vi "String to array.vi"(11 "String":string) -> (2 "Array":dbl[][](array[numeric]))   [LabVIEW 2016]
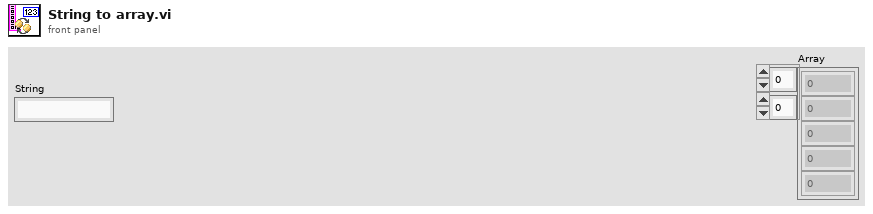
[diagram p1: front panel]
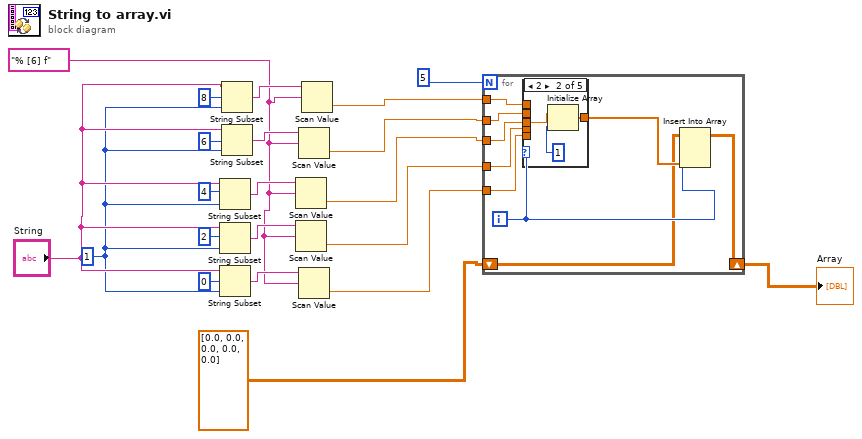
[diagram p0: block diagram]
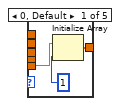
[diagram p2: hidden frame]
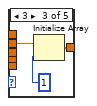
[diagram p3: hidden frame]
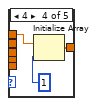
[diagram p4: hidden frame]
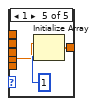
[diagram p5: hidden frame]
diagram:
  w1 = "% [6] f"
  w20 = 1
  n1 = String Subset(string="String", offset (0)=4, length (rest)=w20) -> (substring=w11:string)
  n2 = String Subset(string="String", offset (0)=2, length (rest)=w20) -> (substring=w10:string)
  n3 = String Subset(string="String", offset (0)=0, length (rest)=w20) -> (substring=w8:string)
  n4 = String Subset(string="String", offset (0)=8, length (rest)=w20) -> (substring=w9:string)
  n5 = String Subset(string="String", offset (0)=6, length (rest)=w20) -> (substring=w12:string)
  n6 = Scan Value(string=w11, format string=w1) -> (value=w5:dbl)  [unwired: 1 in, 1 out]
  n7 = Scan Value(string=w10, format string=w1) -> (value=w4:dbl)  [unwired: 1 in, 1 out]
  n8 = Scan Value(string=w12, format string=w1) -> (value=w6:dbl)  [unwired: 1 in, 1 out]
  n9 = Scan Value(string=w8, format string=w1) -> (value=w3:dbl)  [unwired: 1 in, 1 out]
  n10 = Scan Value(string=w9, format string=w1) -> (value=w7:dbl)  [unwired: 1 in, 1 out]
  n11 = for {
    N: 5 -> [_]
    tunnel: w7 -> [w26]
    tunnel: w6 -> [w27]
    tunnel: w5 -> [w28]
    tunnel: w4 -> [w29]
    tunnel: w3 -> [w30]
    shift-right: [w22] -> w14
    shift-left: dbl[][] [[0.0], [0.0], [0.0], [0.0], [0.0]] -> [w23]
    i -> [w25]
    n12 = case shown="2" w25 {
      tunnel: w30 -> [w32 _ _ _ _]
      tunnel: w29 -> [_ _ _ _ w43]
      tunnel: w28 -> [_ w34 _ _ _]
      tunnel: w27 -> [_ _ w37 _ _]
      tunnel: w26 -> [_ _ _ w40 _]
      tunnel: [w31 w35 w38 w41 w44] -> w24
      frame 0, Default {
        n13 = Initialize Array(w32, 1 ("dimension size")) -> (w31:dbl[])
      }
      frame 2 {
        n14 = Initialize Array(w34, 1 ("dimension size")) -> (w35:dbl[])
      }
      frame 3 {
        n15 = Initialize Array(w37, 1 ("dimension size")) -> (w38:dbl[])
      }
      frame 4 {
        n16 = Initialize Array(w40, 1 ("dimension size")) -> (w41:dbl[])
      }
      frame 1 {
        n17 = Initialize Array(w43, 1 ("dimension size")) -> (w44:dbl[])
      }
    }
    n18 = Insert Into Array(array=w23, index (row)=w25, new element=w24) -> (w22:dbl[][])  [unwired: 1 in]
  }
  "Array" <- w14
